vi "12.02.2026.vi"() -> ()   [LabVIEW 2024]
uses:
  <vilib>/Instr/_visa.llb/VISA Configure Serial Port (Instr).vi
panel:
  out "Humidity":dbl(graph)
  out "output 2":dbl
  out "Temperatura":dbl(graph)
  out "output 1":dbl
  out "read buffer":string
  in  "termination char\n(0xA = '\\n' = LF)":u8=10 format="%.0x"
  in  "Operation":dbl
  in  "VISA resource name":refnum<visa-resource-name>
  in  "String":string
  in  "stop":bool
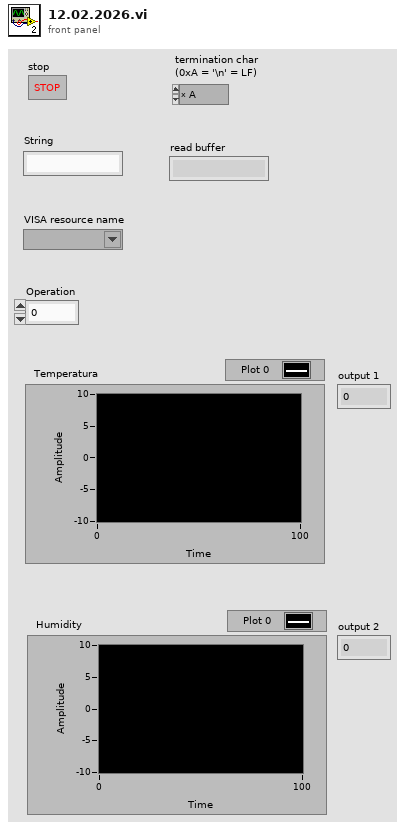
[diagram p1: front panel]
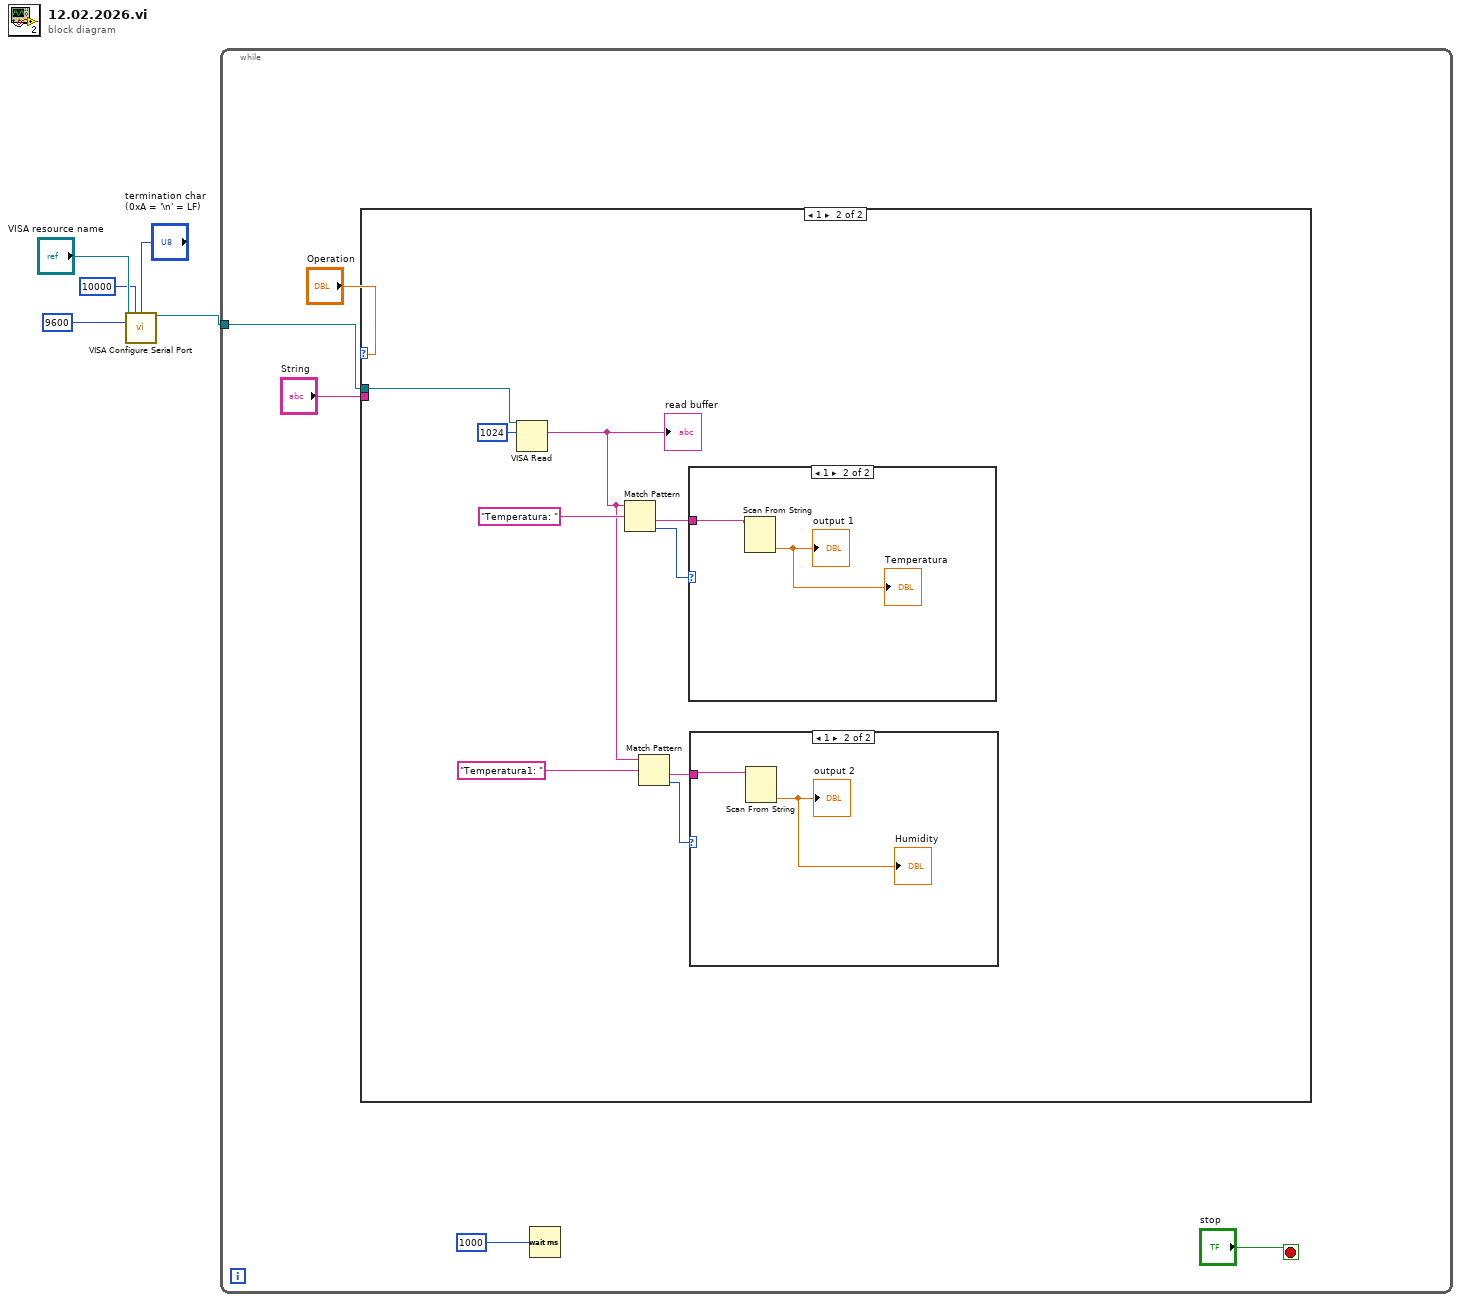
[diagram p0: block diagram]
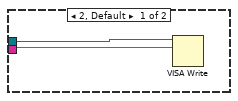
[diagram p2: hidden frame]
diagram:
  n1 = call-poly "VISA Configure Serial Port"("VISA resource name"="VISA resource name", "timeout (10sec)"=u32 10000, "termination char\n(0xA = '\\n' = LF)"="termination char\n(0xA = '\\n' = LF)", "baud rate (9600)"=u32 9600) -> ("VISA resource name out"=w4:refnum<visa-resource-name>)  [unwired: 10 in, 1 out]
  n2 = while {
    tunnel: w4 -> [w8]
    stop <- "stop" stop-if-true
    n3 = case shown="1" "Operation" {
      tunnel: "String" -> [w11 _]
      tunnel: w8 -> [w12 w20]
      frame 2, Default {
        n4 = VISA Write(VISA resource name=w12, write buffer=w11) -> ()  [unwired: 1 in, 3 out]
      }
      frame 1 {
        n5 = VISA Read(VISA resource name=w20, byte count=u32 1024) -> (read buffer=w13:string)  [unwired: 1 in, 3 out]
        "read buffer" <- w13
        n6 = Match Pattern(string=w13, regular expression="Temperatura: ") -> (after substring=w19:string, offset past match=w15:i32)  [unwired: 1 in, 2 out]
        n7 = Match Pattern(string=w13, regular expression="Temperatura1: ") -> (after substring=w16:string, offset past match=w14:i32)  [unwired: 1 in, 2 out]
        n8 = case shown="1" w15 {
          tunnel: w19 -> [_ w25]
          frame 0, Default {
          }
          frame 1 {
            n9 = Scan From String(input string=w25) -> (output 1=→"output 1" →"Temperatura":dbl)  [unwired: 4 in, 3 out]
          }
        }
        n10 = case shown="1" w14 {
          tunnel: w16 -> [_ w23]
          frame 0, Default {
          }
          frame 1 {
            n11 = Scan From String(input string=w23) -> (output 1=→"output 2" →"Humidity":dbl)  [unwired: 4 in, 3 out]
          }
        }
      }
    }
    n12 = Wait (ms)(milliseconds to wait=u32 1000) -> ()  [unwired: 1 out]
  }
